vi "Execute Wash.vi"(8 "Error In":errorcluster, 10 "Car Position Slider":u8(slide) max=3 scale=0.0..4.0, 11 "Data Cluster":T1) -> (0 "Error Out":errorcluster, 3 "Data Cluster Out":T1)   [LabVIEW 2017]
doc: "Execute car wash cycle based on inputs selected\n\n- Check the slider input to match with respective wash options and update UI accordingly\n- Execute timer for reset, read and pause.\n- When cycle completed, pass wait for slider movement to exit position to end car wash"
uses:
  Controls/DataCluster.ctl
  Controls/Wash Options.ctl
  Controls/Car Wash Indicators.ctl
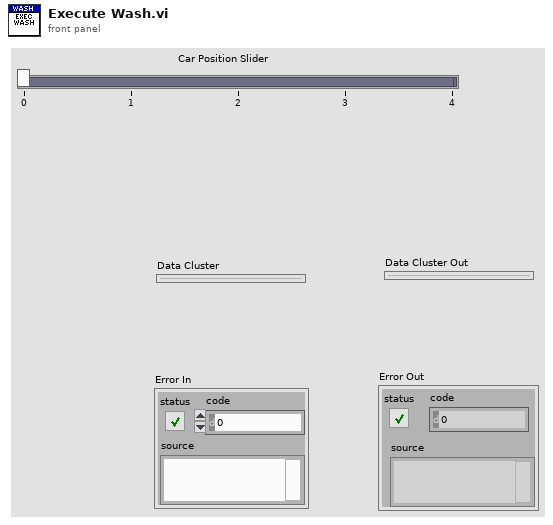
[diagram p1: front panel]
types:
  T1 = typedef "DataCluster.ctl" = cluster{"Wash Options":T2, "Elapsed Time (s)":dbl, "Car Wash Indicators":T3, "Wash Entry":bool, "Wash Running":bool, "Sorted Wash ":enum16{"Under Body Wash", "Bug Remover", "Pre-Soak", "High Pressure Wash", "Low Pressure Wax", "Spot Free Rinse", "Tire Shine Foam", "Air Dry", "Skip"}[], "Timer Elapsed?":bool, "Time Target (s)":dbl}
  T2 = typedef "Wash Options.ctl" = cluster{"Underbody Wash":bool, "Bug Remover":bool, "Pre-Soak":bool, "High Pressure Wash":bool, "Low Pressure Wax":bool, "Spot Free Rinse":bool, "Tire Shine Foam":bool, "Air Dry":bool}
  T3 = typedef "Car Wash Indicators.ctl" = cluster{"Under Body Wash":bool, "Bug Remover":bool, "Pre-Soak":bool, "High Pressure Wash":bool, "Low Pressure Wax":bool, "Spot Free Rinse":bool, "Tire Shine Foam":bool, "Air Dry":bool, "Vehicle Out of Position":bool}
  T4 = enum16{"Under Body Wash", "Bug Remover", "Pre-Soak", "High Pressure Wash", "Low Pressure Wax", "Spot Free Rinse", "Tire Shine Foam", "Air Dry", "Skip"}[]
  T5 = enum16{"Under Body Wash", "Bug Remover", "Pre-Soak", "High Pressure Wash", "Low Pressure Wax", "Spot Free Rinse", "Tire Shine Foam", "Air Dry", "Skip"}
  T6 = enum16{"Create", "Enqueue", "Dequeue", "Enstack", "Flush", "Clear"}
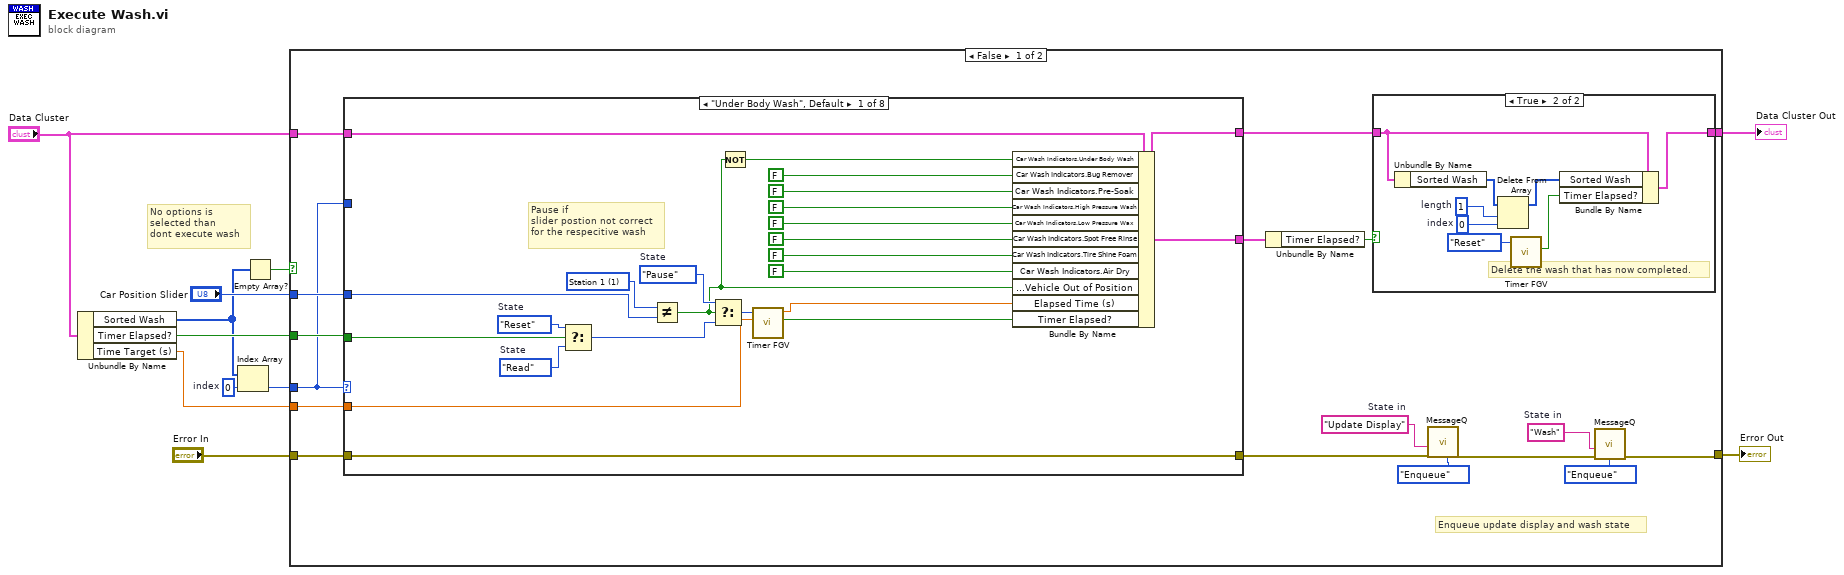
[diagram p0: block diagram]
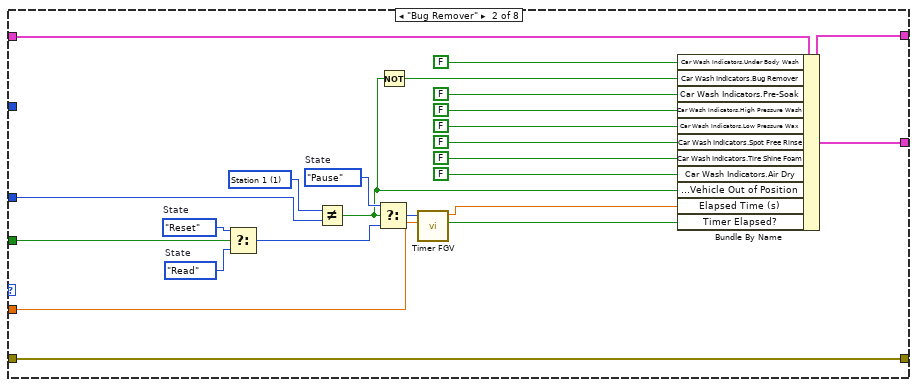
[diagram p3: hidden frame]
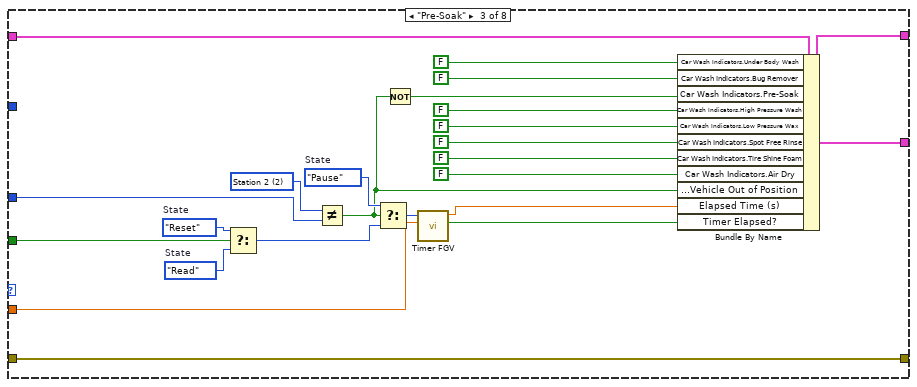
[diagram p4: hidden frame]
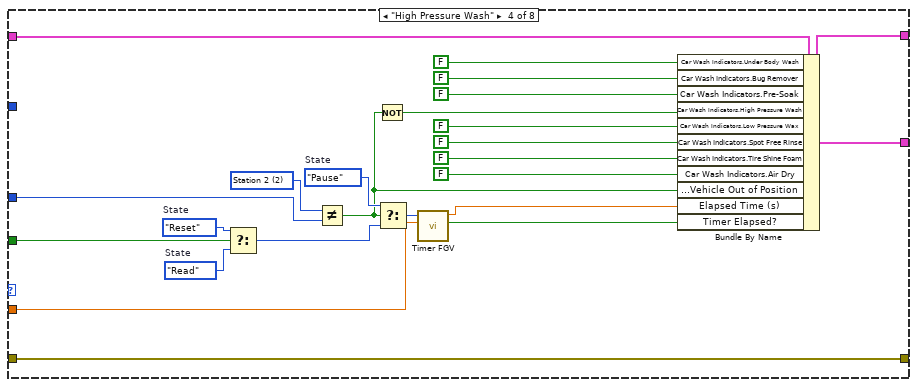
[diagram p5: hidden frame]
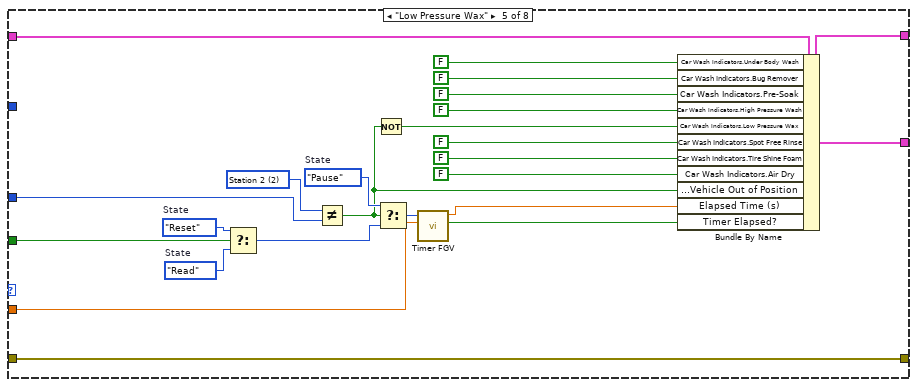
[diagram p6: hidden frame]
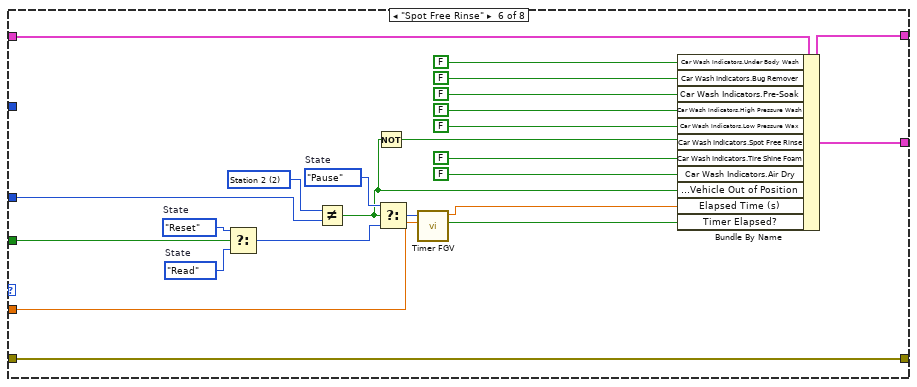
[diagram p7: hidden frame]
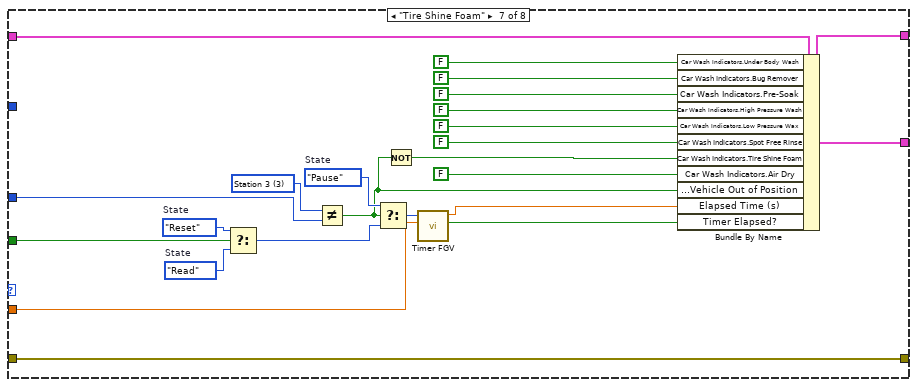
[diagram p8: hidden frame]
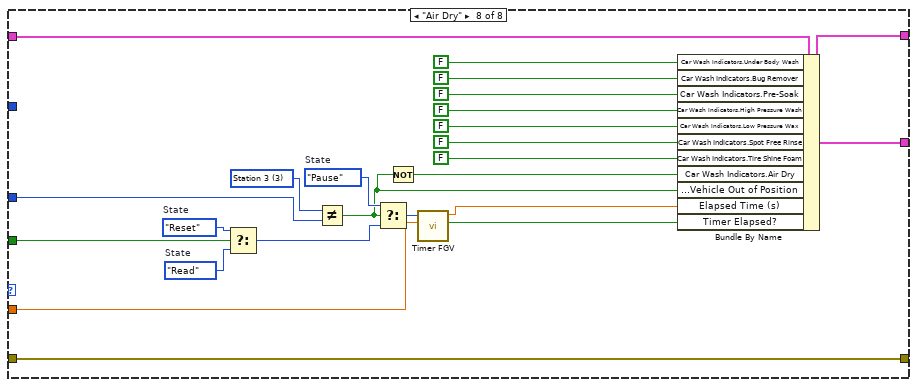
[diagram p9: hidden frame]
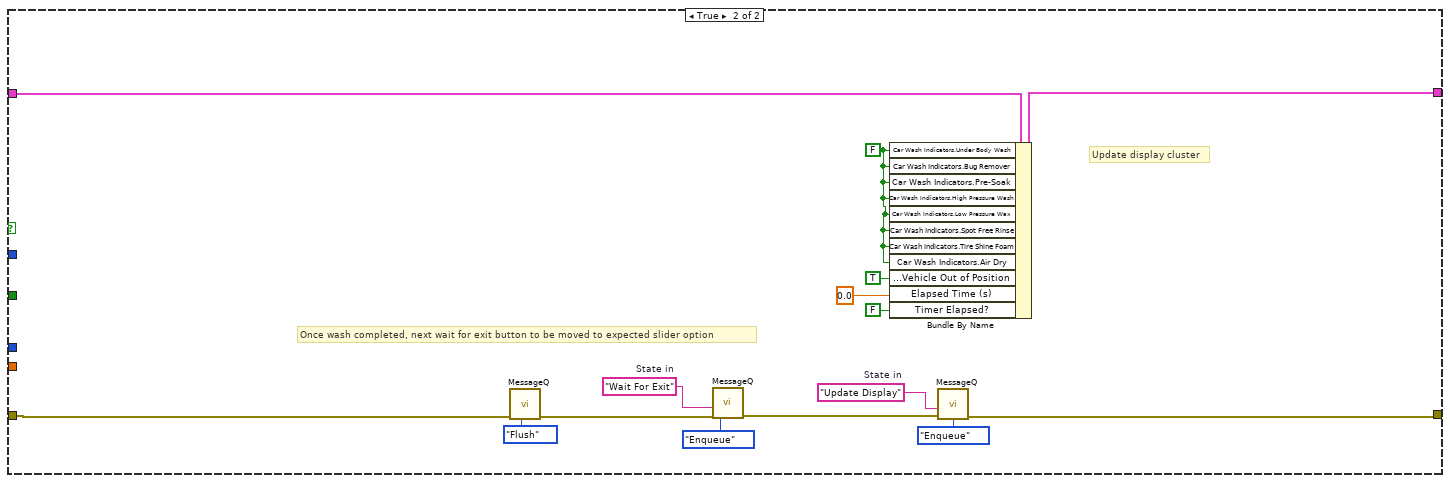
[diagram p10: hidden frame]
diagram:
  w8 = 0  # index
  # "No options is selected than\ndont execute wash"
  n1 = Unbundle By Name("Data Cluster") -> ("Sorted Wash"=w4:T4, "Timer Elapsed?"=w10:bool, "Time Target (s)"=w6:dbl)
  n2 = Index Array(array=w4, index=w8) -> (element=w7:T5)
  n3 = Empty Array?(array=w4) -> (empty?=w3:bool)
  n4 = case shown="False" w3 {
    tunnel: "Data Cluster" -> [w28 w232]
    tunnel: w10 -> [w27 _]
    tunnel: "Car Position Slider" -> [w26 _]
    tunnel: w7 -> [w25 _]
    tunnel: w6 -> [w24 _]
    tunnel: [w20 w231] -> w5
    tunnel: "Error In" -> [w13 w227]
    tunnel: [w14 w222] -> w1
    frame False {
      w16 = "Wash"  # State in
      w17 = "Update Display"  # State in
      # "Enqueue update display and wash state"
      n5 = case shown="\"Under Body Wash\", Default" w25 {
        tunnel: w28 -> [w60 w83 w106 w129 w152 w175 w198 w221]
        tunnel: w27 -> [w52 w75 w98 w121 w144 w167 w190 w213]
        tunnel: [w41 w64 w87 w110 w133 w156 w179 w202] -> w23
        tunnel: w26 -> [w48 w71 w94 w117 w140 w163 w186 w209]
        tunnel: w25 -> [_ _ _ _ _ _ _ _]
        tunnel: w24 -> [w42 w65 w88 w111 w134 w157 w181 w204]
        tunnel: [w41 w64 w87 w110 w133 w156 w179 w202] -> w21
        tunnel: w13 -> [w40 w63 w86 w109 w132 w155 w178 w201]
        tunnel: [w40 w63 w86 w109 w132 w155 w178 w201] -> w12
        frame "Under Body Wash", Default {
          w43 = u8 1 items=["Entry", "Station 1", "Station 2", "Station 3", "Exit"] ("Car Position Slider 2")
          w47 = enum16{"Reset", "Read", "Pause"}."Pause"  # State
          w50 = enum16{"Reset", "Read", "Pause"}."Read"  # State
          w51 = enum16{"Reset", "Read", "Pause"}."Reset"  # State
          # "Pause if \nslider postion not correct\nfor the respecitive wash"
          n6 = Select(t=w51, s=w52, f=w50) -> (s? t:f=w49:enum16{"Reset", "Read", "Pause"})
          n7 = Not Equal?(x=w43, y=w48) -> (x != y?=w39:bool)
          n8 = Select(t=w47, s=w39, f=w49) -> (s? t:f=w46:enum16{"Reset", "Read", "Pause"})
          n9 = Not(x=w39) -> (.not. x?=w38:bool)
          n10 = call "Timer FGV.vi"("Time Target"=w42, "State"=w46) -> ("Time Elapsed"=w44:bool, "Elapsed Time"=w45:dbl)  [unwired: 7 in, 1 out]
          n11 = Bundle By Name(cluster=w60, "Car Wash Indicators.Under Body Wash"=w38, "Car Wash Indicators.Bug Remover"=FALSE ("Car Wash Indicators.Under Body Wash"), "Car Wash Indicators.Pre-Soak"=FALSE ("Car Wash Indicators.Under Body Wash"), "Car Wash Indicators.High Pressure Wash"=FALSE ("Car Wash Indicators.Under Body Wash"), "Car Wash Indicators.Low Pressure Wax"=FALSE ("Car Wash Indicators.Under Body Wash"), "Car Wash Indicators.Spot Free Rinse"=FALSE ("Car Wash Indicators.Under Body Wash"), "Car Wash Indicators.Tire Shine Foam"=FALSE ("Car Wash Indicators.Under Body Wash"), "Car Wash Indicators.Air Dry"=FALSE ("Car Wash Indicators.Under Body Wash"), "Car Wash Indicators.Vehicle Out of Position"=w39, "Elapsed Time (s)"=w45, "Timer Elapsed?"=w44) -> (w41:T1)
        }
        frame "Bug Remover" {
          w66 = u8 1 items=["Entry", "Station 1", "Station 2", "Station 3", "Exit"] ("Car Position Slider 2")
          w70 = enum16{"Reset", "Read", "Pause"}."Pause"  # State
          w73 = enum16{"Reset", "Read", "Pause"}."Read"  # State
          w74 = enum16{"Reset", "Read", "Pause"}."Reset"  # State
          n12 = Select(t=w74, s=w75, f=w73) -> (s? t:f=w72:enum16{"Reset", "Read", "Pause"})
          n13 = Not Equal?(x=w66, y=w71) -> (x != y?=w62:bool)
          n14 = Select(t=w70, s=w62, f=w72) -> (s? t:f=w69:enum16{"Reset", "Read", "Pause"})
          n15 = Not(x=w62) -> (.not. x?=w61:bool)
          n16 = call "Timer FGV.vi"("Time Target"=w65, "State"=w69) -> ("Time Elapsed"=w67:bool, "Elapsed Time"=w68:dbl)  [unwired: 7 in, 1 out]
          n17 = Bundle By Name(cluster=w83, "Car Wash Indicators.Under Body Wash"=FALSE, "Car Wash Indicators.Bug Remover"=w61, "Car Wash Indicators.Pre-Soak"=FALSE ("Car Wash Indicators.Under Body Wash"), "Car Wash Indicators.High Pressure Wash"=FALSE ("Car Wash Indicators.Under Body Wash"), "Car Wash Indicators.Low Pressure Wax"=FALSE ("Car Wash Indicators.Under Body Wash"), "Car Wash Indicators.Spot Free Rinse"=FALSE ("Car Wash Indicators.Under Body Wash"), "Car Wash Indicators.Tire Shine Foam"=FALSE ("Car Wash Indicators.Under Body Wash"), "Car Wash Indicators.Air Dry"=FALSE ("Car Wash Indicators.Under Body Wash"), "Car Wash Indicators.Vehicle Out of Position"=w62, "Elapsed Time (s)"=w68, "Timer Elapsed?"=w67) -> (w64:T1)
        }
        frame "Pre-Soak" {
          w89 = u8 2 items=["Entry", "Station 1", "Station 2", "Station 3", "Exit"] ("Car Position Slider 2")
          w93 = enum16{"Reset", "Read", "Pause"}."Pause"  # State
          w96 = enum16{"Reset", "Read", "Pause"}."Read"  # State
          w97 = enum16{"Reset", "Read", "Pause"}."Reset"  # State
          n18 = Select(t=w97, s=w98, f=w96) -> (s? t:f=w95:enum16{"Reset", "Read", "Pause"})
          n19 = Not Equal?(x=w89, y=w94) -> (x != y?=w85:bool)
          n20 = Select(t=w93, s=w85, f=w95) -> (s? t:f=w92:enum16{"Reset", "Read", "Pause"})
          n21 = Not(x=w85) -> (.not. x?=w84:bool)
          n22 = call "Timer FGV.vi"("Time Target"=w88, "State"=w92) -> ("Time Elapsed"=w90:bool, "Elapsed Time"=w91:dbl)  [unwired: 7 in, 1 out]
          n23 = Bundle By Name(cluster=w106, "Car Wash Indicators.Under Body Wash"=FALSE, "Car Wash Indicators.Bug Remover"=FALSE ("Car Wash Indicators.Under Body Wash"), "Car Wash Indicators.Pre-Soak"=w84, "Car Wash Indicators.High Pressure Wash"=FALSE ("Car Wash Indicators.Under Body Wash"), "Car Wash Indicators.Low Pressure Wax"=FALSE ("Car Wash Indicators.Under Body Wash"), "Car Wash Indicators.Spot Free Rinse"=FALSE ("Car Wash Indicators.Under Body Wash"), "Car Wash Indicators.Tire Shine Foam"=FALSE ("Car Wash Indicators.Under Body Wash"), "Car Wash Indicators.Air Dry"=FALSE ("Car Wash Indicators.Under Body Wash"), "Car Wash Indicators.Vehicle Out of Position"=w85, "Elapsed Time (s)"=w91, "Timer Elapsed?"=w90) -> (w87:T1)
        }
        frame "High Pressure Wash" {
          w112 = u8 2 items=["Entry", "Station 1", "Station 2", "Station 3", "Exit"] ("Car Position Slider 2")
          w116 = enum16{"Reset", "Read", "Pause"}."Pause"  # State
          w119 = enum16{"Reset", "Read", "Pause"}."Read"  # State
          w120 = enum16{"Reset", "Read", "Pause"}."Reset"  # State
          n24 = Select(t=w120, s=w121, f=w119) -> (s? t:f=w118:enum16{"Reset", "Read", "Pause"})
          n25 = Not Equal?(x=w112, y=w117) -> (x != y?=w108:bool)
          n26 = Not(x=w108) -> (.not. x?=w107:bool)
          n27 = Select(t=w116, s=w108, f=w118) -> (s? t:f=w115:enum16{"Reset", "Read", "Pause"})
          n28 = call "Timer FGV.vi"("Time Target"=w111, "State"=w115) -> ("Time Elapsed"=w113:bool, "Elapsed Time"=w114:dbl)  [unwired: 7 in, 1 out]
          n29 = Bundle By Name(cluster=w129, "Car Wash Indicators.Under Body Wash"=FALSE, "Car Wash Indicators.Bug Remover"=FALSE ("Car Wash Indicators.Under Body Wash"), "Car Wash Indicators.Pre-Soak"=FALSE ("Car Wash Indicators.Under Body Wash"), "Car Wash Indicators.High Pressure Wash"=w107, "Car Wash Indicators.Low Pressure Wax"=FALSE ("Car Wash Indicators.Under Body Wash"), "Car Wash Indicators.Spot Free Rinse"=FALSE ("Car Wash Indicators.Under Body Wash"), "Car Wash Indicators.Tire Shine Foam"=FALSE ("Car Wash Indicators.Under Body Wash"), "Car Wash Indicators.Air Dry"=FALSE ("Car Wash Indicators.Under Body Wash"), "Car Wash Indicators.Vehicle Out of Position"=w108, "Elapsed Time (s)"=w114, "Timer Elapsed?"=w113) -> (w110:T1)
        }
        frame "Low Pressure Wax" {
          w135 = u8 2 items=["Entry", "Station 1", "Station 2", "Station 3", "Exit"] ("Car Position Slider 2")
          w139 = enum16{"Reset", "Read", "Pause"}."Pause"  # State
          w142 = enum16{"Reset", "Read", "Pause"}."Read"  # State
          w143 = enum16{"Reset", "Read", "Pause"}."Reset"  # State
          n30 = Select(t=w143, s=w144, f=w142) -> (s? t:f=w141:enum16{"Reset", "Read", "Pause"})
          n31 = Not Equal?(x=w135, y=w140) -> (x != y?=w131:bool)
          n32 = Not(x=w131) -> (.not. x?=w130:bool)
          n33 = Select(t=w139, s=w131, f=w141) -> (s? t:f=w138:enum16{"Reset", "Read", "Pause"})
          n34 = call "Timer FGV.vi"("Time Target"=w134, "State"=w138) -> ("Time Elapsed"=w136:bool, "Elapsed Time"=w137:dbl)  [unwired: 7 in, 1 out]
          n35 = Bundle By Name(cluster=w152, "Car Wash Indicators.Under Body Wash"=FALSE, "Car Wash Indicators.Bug Remover"=FALSE ("Car Wash Indicators.Under Body Wash"), "Car Wash Indicators.Pre-Soak"=FALSE ("Car Wash Indicators.Under Body Wash"), "Car Wash Indicators.High Pressure Wash"=FALSE ("Car Wash Indicators.Under Body Wash"), "Car Wash Indicators.Low Pressure Wax"=w130, "Car Wash Indicators.Spot Free Rinse"=FALSE ("Car Wash Indicators.Under Body Wash"), "Car Wash Indicators.Tire Shine Foam"=FALSE ("Car Wash Indicators.Under Body Wash"), "Car Wash Indicators.Air Dry"=FALSE ("Car Wash Indicators.Under Body Wash"), "Car Wash Indicators.Vehicle Out of Position"=w131, "Elapsed Time (s)"=w137, "Timer Elapsed?"=w136) -> (w133:T1)
        }
        frame "Spot Free Rinse" {
          w158 = u8 2 items=["Entry", "Station 1", "Station 2", "Station 3", "Exit"] ("Car Position Slider 2")
          w162 = enum16{"Reset", "Read", "Pause"}."Pause"  # State
          w165 = enum16{"Reset", "Read", "Pause"}."Read"  # State
          w166 = enum16{"Reset", "Read", "Pause"}."Reset"  # State
          n36 = Select(t=w166, s=w167, f=w165) -> (s? t:f=w164:enum16{"Reset", "Read", "Pause"})
          n37 = Not Equal?(x=w158, y=w163) -> (x != y?=w154:bool)
          n38 = Not(x=w154) -> (.not. x?=w153:bool)
          n39 = Select(t=w162, s=w154, f=w164) -> (s? t:f=w161:enum16{"Reset", "Read", "Pause"})
          n40 = call "Timer FGV.vi"("Time Target"=w157, "State"=w161) -> ("Time Elapsed"=w159:bool, "Elapsed Time"=w160:dbl)  [unwired: 7 in, 1 out]
          n41 = Bundle By Name(cluster=w175, "Car Wash Indicators.Under Body Wash"=FALSE, "Car Wash Indicators.Bug Remover"=FALSE ("Car Wash Indicators.Under Body Wash"), "Car Wash Indicators.Pre-Soak"=FALSE ("Car Wash Indicators.Under Body Wash"), "Car Wash Indicators.High Pressure Wash"=FALSE ("Car Wash Indicators.Under Body Wash"), "Car Wash Indicators.Low Pressure Wax"=FALSE ("Car Wash Indicators.Under Body Wash"), "Car Wash Indicators.Spot Free Rinse"=w153, "Car Wash Indicators.Tire Shine Foam"=FALSE ("Car Wash Indicators.Under Body Wash"), "Car Wash Indicators.Air Dry"=FALSE ("Car Wash Indicators.Under Body Wash"), "Car Wash Indicators.Vehicle Out of Position"=w154, "Elapsed Time (s)"=w160, "Timer Elapsed?"=w159) -> (w156:T1)
        }
        frame "Tire Shine Foam" {
          w180 = u8 3 items=["Entry", "Station 1", "Station 2", "Station 3", "Exit"] ("Car Position Slider 2")
          w185 = enum16{"Reset", "Read", "Pause"}."Pause"  # State
          w188 = enum16{"Reset", "Read", "Pause"}."Read"  # State
          w189 = enum16{"Reset", "Read", "Pause"}."Reset"  # State
          n42 = Select(t=w189, s=w190, f=w188) -> (s? t:f=w187:enum16{"Reset", "Read", "Pause"})
          n43 = Not Equal?(x=w180, y=w186) -> (x != y?=w177:bool)
          n44 = Select(t=w185, s=w177, f=w187) -> (s? t:f=w184:enum16{"Reset", "Read", "Pause"})
          n45 = Not(x=w177) -> (.not. x?=w176:bool)
          n46 = call "Timer FGV.vi"("Time Target"=w181, "State"=w184) -> ("Time Elapsed"=w182:bool, "Elapsed Time"=w183:dbl)  [unwired: 7 in, 1 out]
          n47 = Bundle By Name(cluster=w198, "Car Wash Indicators.Under Body Wash"=FALSE, "Car Wash Indicators.Bug Remover"=FALSE ("Car Wash Indicators.Under Body Wash"), "Car Wash Indicators.Pre-Soak"=FALSE ("Car Wash Indicators.Under Body Wash"), "Car Wash Indicators.High Pressure Wash"=FALSE ("Car Wash Indicators.Under Body Wash"), "Car Wash Indicators.Low Pressure Wax"=FALSE ("Car Wash Indicators.Under Body Wash"), "Car Wash Indicators.Spot Free Rinse"=FALSE ("Car Wash Indicators.Under Body Wash"), "Car Wash Indicators.Tire Shine Foam"=w176, "Car Wash Indicators.Air Dry"=FALSE ("Car Wash Indicators.Under Body Wash"), "Car Wash Indicators.Vehicle Out of Position"=w177, "Elapsed Time (s)"=w183, "Timer Elapsed?"=w182) -> (w179:T1)
        }
        frame "Air Dry" {
          w205 = u8 3 items=["Entry", "Station 1", "Station 2", "Station 3", "Exit"] ("Car Position Slider 2")
          w208 = enum16{"Reset", "Read", "Pause"}."Pause"  # State
          w211 = enum16{"Reset", "Read", "Pause"}."Read"  # State
          w212 = enum16{"Reset", "Read", "Pause"}."Reset"  # State
          n48 = Select(t=w212, s=w213, f=w211) -> (s? t:f=w210:enum16{"Reset", "Read", "Pause"})
          n49 = Not Equal?(x=w205, y=w209) -> (x != y?=w200:bool)
          n50 = Select(t=w208, s=w200, f=w210) -> (s? t:f=w207:enum16{"Reset", "Read", "Pause"})
          n51 = Not(x=w200) -> (.not. x?=w199:bool)
          n52 = call "Timer FGV.vi"("Time Target"=w204, "State"=w207) -> ("Time Elapsed"=w203:bool, "Elapsed Time"=w206:dbl)  [unwired: 7 in, 1 out]
          n53 = Bundle By Name(cluster=w221, "Car Wash Indicators.Under Body Wash"=FALSE, "Car Wash Indicators.Bug Remover"=FALSE ("Car Wash Indicators.Under Body Wash"), "Car Wash Indicators.Pre-Soak"=FALSE ("Car Wash Indicators.Under Body Wash"), "Car Wash Indicators.High Pressure Wash"=FALSE ("Car Wash Indicators.Under Body Wash"), "Car Wash Indicators.Low Pressure Wax"=FALSE ("Car Wash Indicators.Under Body Wash"), "Car Wash Indicators.Spot Free Rinse"=FALSE ("Car Wash Indicators.Under Body Wash"), "Car Wash Indicators.Tire Shine Foam"=FALSE ("Car Wash Indicators.Under Body Wash"), "Car Wash Indicators.Air Dry"=w199, "Car Wash Indicators.Vehicle Out of Position"=w200, "Elapsed Time (s)"=w206, "Timer Elapsed?"=w203) -> (w202:T1)
        }
      }
      n54 = Unbundle By Name(w23) -> ("Timer Elapsed?"=w22:bool)
      n55 = case shown="True" w22 {
        tunnel: w21 -> [w29 w34]
        tunnel: [w29 w33] -> w20
        frame False {
        }
        frame True {
          w35 = 1  # length
          w36 = 0  # index
          # "Delete the wash that has now completed."
          n56 = Unbundle By Name(w34) -> ("Sorted Wash"=w37:T4)
          n57 = Delete From Array(array=w37, length=w35, index=w36) -> (array with subset deleted=w32:T4)  [unwired: 1 out]
          n58 = call "Timer FGV.vi"("State"=enum16{"Reset", "Read", "Pause"}."Reset") -> ("Time Elapsed"=w30:bool)  [unwired: 8 in, 2 out]
          n59 = Bundle By Name(cluster=w34, "Sorted Wash"=w32, "Timer Elapsed?"=w30) -> (w33:T1)
        }
      }
      n60 = call "MessageQ.vi"("Error In"=w12, "State in"=w17, "QState"=T6."Enqueue") -> ("Error Out"=w15:errorcluster)  [unwired: 7 in, 1 out]
      n61 = call "MessageQ.vi"("Error In"=w15, "State in"=w16, "QState"=T6."Enqueue") -> ("Error Out"=w14:errorcluster)  [unwired: 7 in, 1 out]
    }
    frame True {
      w224 = "Update Display"  # State in
      w230 = "Wait For Exit"  # State in
      w235 = FALSE ("Car Wash Indicators.Under Body Wash")
      # "Update display cluster"
      # "Once wash completed, next wait for exit button to be moved to expected slider option"
      n62 = call "MessageQ.vi"("Error In"=w227, "QState"=T6."Flush") -> ("Error Out"=w226:errorcluster)  [unwired: 8 in, 1 out]
      n63 = call "MessageQ.vi"("Error In"=w226, "State in"=w230, "QState"=T6."Enqueue") -> ("Error Out"=w223:errorcluster)  [unwired: 7 in, 1 out]
      n64 = Bundle By Name(cluster=w232, "Car Wash Indicators.Under Body Wash"=w235, "Car Wash Indicators.Bug Remover"=w235, "Car Wash Indicators.Pre-Soak"=w235, "Car Wash Indicators.High Pressure Wash"=w235, "Car Wash Indicators.Low Pressure Wax"=w235, "Car Wash Indicators.Spot Free Rinse"=w235, "Car Wash Indicators.Tire Shine Foam"=w235, "Car Wash Indicators.Air Dry"=w235, "Car Wash Indicators.Vehicle Out of Position"=TRUE, "Elapsed Time (s)"=0.0 ("Elapsed Time"), "Timer Elapsed?"=FALSE) -> (w231:T1)
      n65 = call "MessageQ.vi"("Error In"=w223, "State in"=w224, "QState"=T6."Enqueue") -> ("Error Out"=w222:errorcluster)  [unwired: 7 in, 1 out]
    }
  }
  "Data Cluster Out" <- w5
  "Error Out" <- w1
